vi "Image Tester.vi"(11 "Particle Report":T1) -> (3 "Positive":bool)   [LabVIEW 2016]
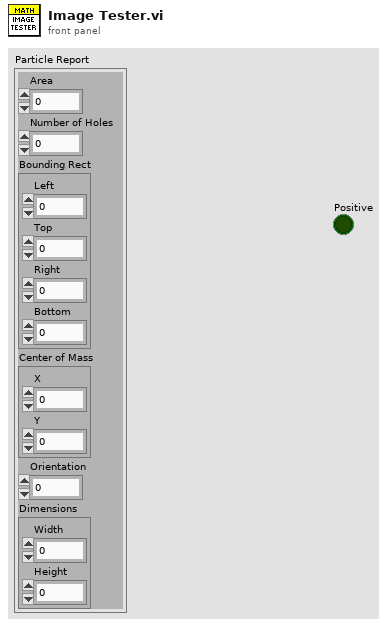
[diagram p1: front panel]
types:
  T1 = cluster{"Area":dbl, "Number of Holes":dbl, "Bounding Rect":cluster{"Left":dbl, "Top":dbl, "Right":dbl, "Bottom":dbl}, "Center of Mass":cluster{"X":dbl, "Y":dbl}, "Orientation":dbl, "Dimensions":cluster{"Width":dbl, "Height":dbl}}
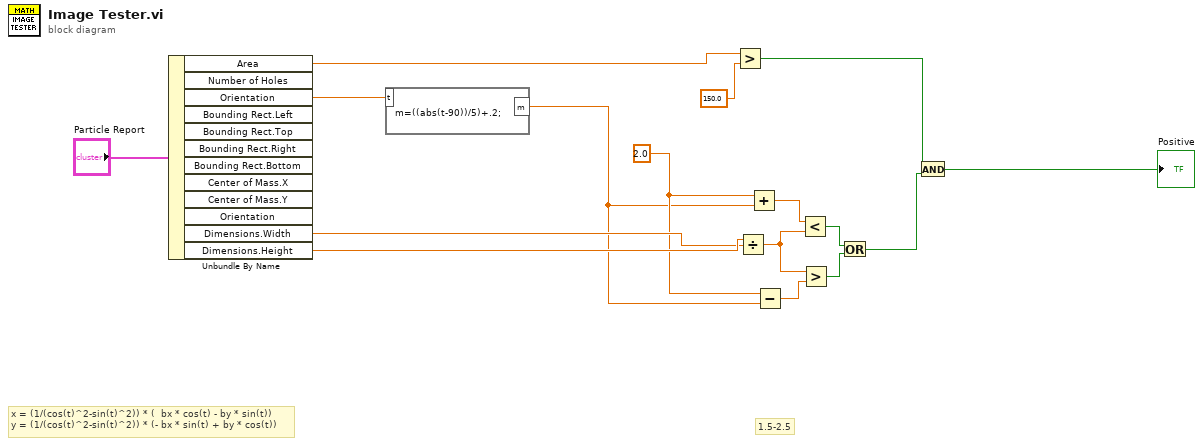
[diagram p0: block diagram]
diagram:
  w5 = 2.0
  # "x = (1/(cos(t)^2-sin(t)^2)) * (  bx * cos(t) - by * sin(t))\ny = (1/(cos(t)^2-sin(t)^2)) * (- bx * sin(t) + by * cos(t))"
  # "1.5-2.5"
  n1 = Unbundle By Name("Particle Report") -> ("Area"=w8:dbl, "Orientation"=w1:dbl, "Dimensions.Width"=w6:dbl, "Dimensions.Height"=w7:dbl)  [unwired: 8 out]
  n2 = formula code="m=((abs(t-90))/5)+.2;"("t"=w1) -> ("m"=w2:dbl)
  n3 = Greater?(x=w8, y=150.0 ("x")) -> (0:w12:bool)
  n4 = Divide(x=w7, y=w6) -> (x/y=w13:dbl)
  n5 = Add(x=w5, y=w2) -> (x+y=w3:dbl)
  n6 = Subtract(x=w5, y=w2) -> (x-y=w4:dbl)
  n7 = Less?(x=w3, y=w13) -> (x < y?=w15:bool)
  n8 = Greater?(x=w13, y=w4) -> (0:w14:bool)
  n9 = Or(x=w15, y=w14) -> (x .or. y?=w11:bool)
  n10 = And(x=w12, y=w11) -> (x .and. y?=→"Positive":bool)
